vi "Read UI config file.vi"(8 "error in (no error)":errorcluster) -> (0 "error out":errorcluster, 3 "output cluster":T1={"Font"="Consolas", "Font Size"=0, "BG Color"=0, "Text Color"=0, "Debug?"=FALSE})   [LabVIEW 2023, in "VeriStand Console.lvlib"]
uses:
  VeriStand Console.lvlib
  TypeDefs/UI Settings.ctl
  <vilib>/Utility/config.llb/Read Key (String).vi
  <vilib>/Utility/config.llb/Read Key (U32).vi
  <vilib>/Utility/config.llb/Read Key (Boolean).vi
  <vilib>/Utility/config.llb/NI_LVConfig.lvlib
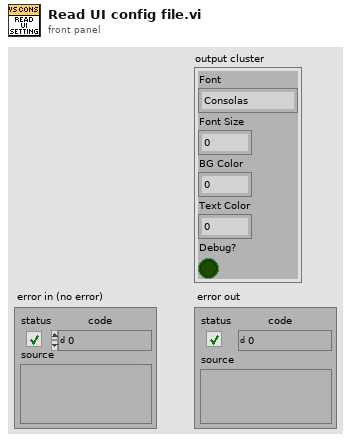
[diagram p1: front panel]
types:
  T1 = typedef "VeriStand Console.lvlib/UI Settings.ctl" = cluster{"Font":string, "Font Size":u32, "BG Color":u32, "Text Color":u32, "Debug?":bool}
  T2 = typedef "NI_LVConfig.lvlib/Config Data RefNum.ctl" = refnum<k1>
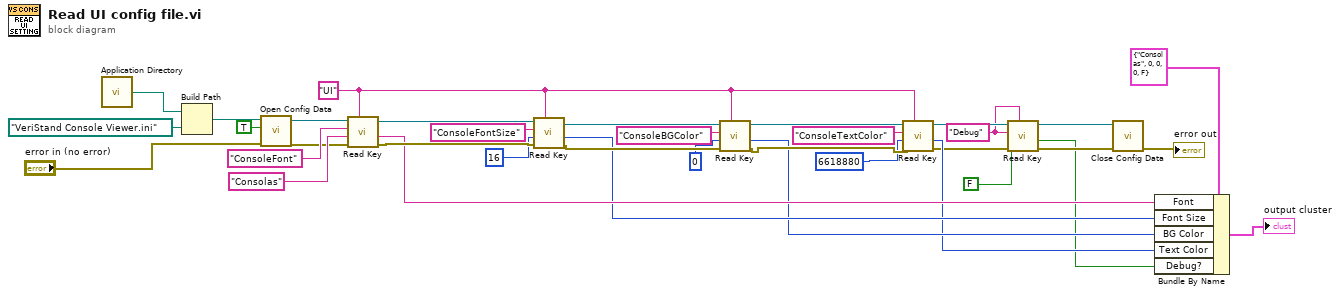
[diagram p0: block diagram]
diagram:
  w3 = "Debug" ("key")
  w33 = "UI" ("section")
  n1 = call <vilib>:"Application Directory.vi"() -> ("Application Directory"=w16:path)
  n2 = Build Path(base path=w16, name or relative path=path "VeriStand Console Viewer.ini") -> (appended path=w17:path)
  n3 = call <vilib>:"Open Config Data.vi"("error in (no error)"="error in (no error)", "create file if necessary (T)"=TRUE, "configuration file path"=w17) -> ("error out"=w21:errorcluster, "refnum"=w20:T2)  [unwired: 6 in, 1 out]
  n4 = call-poly <vilib>:"Read Key.vi"("section"=w33, "error in (no error)"=w21, "default value"="Consolas", "key"="ConsoleFont", "refnum"=w20) -> ("error out"=w34:errorcluster, "value"=w14:string, "refnum out"=w24:T2)  [unwired: 3 in, 1 out]
  n5 = call-poly <vilib>:"Read Key.vi"("section"=w33, "error in (no error)"=w34, "default value"=u32 16, "key"="ConsoleFontSize", "refnum"=w24) -> ("error out"=w35:errorcluster, "value"=w13:u32, "refnum out"=w32:T2)  [unwired: 3 in, 1 out]
  n6 = call-poly <vilib>:"Read Key.vi"("section"=w33, "error in (no error)"=w35, "default value"=u32 0, "key"="ConsoleBGColor", "refnum"=w32) -> ("error out"=w36:errorcluster, "value"=w12:u32, "refnum out"=w31:T2)  [unwired: 3 in, 1 out]
  n7 = call-poly <vilib>:"Read Key.vi"("section"=w33, "error in (no error)"=w36, "default value"=u32 6618880, "key"="ConsoleTextColor", "refnum"=w31) -> ("error out"=w8:errorcluster, "value"=w11:u32, "refnum out"=w5:T2)  [unwired: 3 in, 1 out]
  n8 = call-poly <vilib>:"Read Key.vi"("section"=w3, "error in (no error)"=w8, "default value"=FALSE, "key"=w3, "refnum"=w5) -> ("error out"=w6:errorcluster, "value"=w1:bool, "refnum out"=w4:T2)  [unwired: 3 in, 1 out]
  n9 = call <vilib>:"Close Config Data.vi"("error in (no error)"=w6, "refnum"=w4) -> ("error out"=→"error out":errorcluster)  [unwired: 8 in, 1 out]
  n10 = Bundle By Name(cluster=T1 {"Font"="Consolas", "Font Size"=0, "BG Color"=0, "Text Color"=0, "Debug?"=FALSE}, "Font"=w14, "Font Size"=w13, "BG Color"=w12, "Text Color"=w11, "Debug?"=w1) -> (→"output cluster":T1)
